vi "Cond Attr Get Clock.vi"(8 "error in (no error)":errorcluster, 11 "Cond Attr in":T2) -> (0 "error out":errorcluster, 2 "clock id":T1=enum."Monotonic", 3 "Cond Attr out":T2)   [LabVIEW 2016, in "Linux RT IPC.POSIX Threads.lvlib" / "Cond Attr.lvclass"]
doc: "Calls pthread_condattr_getclock() on the pthread cond attribute object encapsulated by Cond Attr.\n\nThis VI returns the current clock that the conditional variable is configured to use for timeout evaluation.\n\nRefer to online POSIX documentation for more information."
uses:
  Cond Attr.lvclass
  Controls/reference.ctl
  C:/Git/SourceTree/LinuxRT-IPC/Source/POSIX Threads/Classes/POSIX Thread Object/POSIX Thread Object.lvclass
  <vilib>/NI/NI Linux RT Utilities/Controls/Public/C Enums/clockid_t.ctl
  POSIX Thread Object/POSIX Thread Object.lvclass/POSIX Thread Object.ctl
  POSIX Thread Object/Private VIs/libpthread path.vi
  POSIX Thread Object/Private VIs/get pthread error.vi
  POSIX Thread Object/POSIX Thread Object.lvclass
  <vilib>/NI/NI Linux RT Utilities/Linux RT Utilities.lvlib
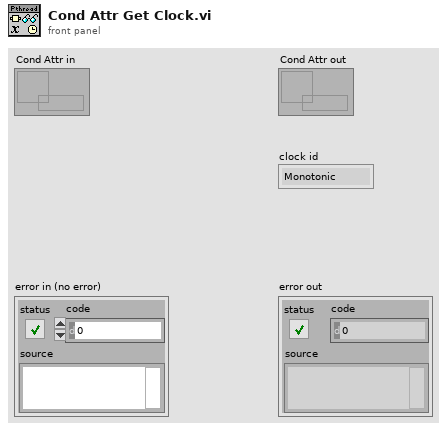
[diagram p1: front panel]
types:
  T1 = typedef "Linux RT Utilities.lvlib/clockid_t.ctl" = enum16{"Realtime", "Monotonic"}
  T2 = typedef "Linux RT IPC.POSIX Threads.lvlib/Cond Attr.lvclass/reference.ctl" = refnum<data-value>
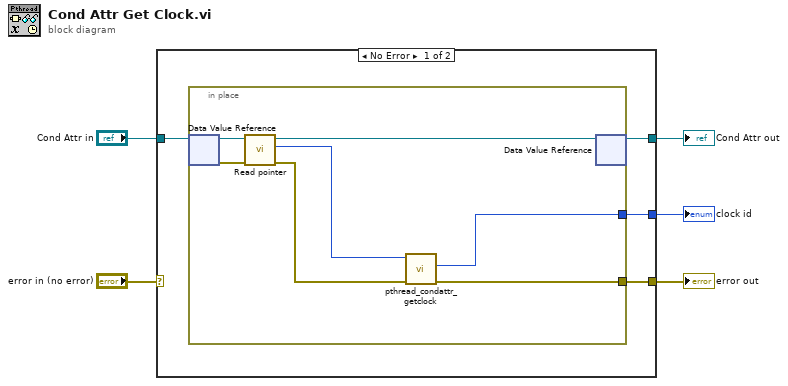
[diagram p0: block diagram]
diagram:
  n1 = case shown="No Error" "error in (no error)" {
    selector: "error in (no error)" -> [_ w18]
    tunnel: [w7 w18] -> w4
    tunnel: "Cond Attr in" -> [w9 w17]
    tunnel: [w8 w17] -> w2
    tunnel: [w6 _] -> w1
    frame No Error {
      n2 = in-place {
        in-place-border: [w12] -> w7
        in-place-border: [w10] -> w6
        n3 = in-place-dvr #1(w9) -> (w16:refnum<class "Cond Attr.lvclass">, w14:errorcluster)
        n4 = call "Read pointer.vi"("error in (no error)"=w14, "POSIX Thread Object in"=w16) -> ("error out"=w13:errorcluster, "pointer"=w11:u64, "POSIX Thread Object out"=w15:refnum<class "Cond Attr.lvclass">)  [unwired: 7 in]
        n5 = call "pthread_condattr_getclock.vi"("error in (no error)"=w13, "cond attr ptr in"=w11) -> ("error out"=w12:errorcluster, "clock id"=w10:T1)  [unwired: 7 in, 1 out]
        n6 = in-place-dvr #1(w15) -> (w8:T2)  [unwired: 1 out]
      }
    }
    frame Error {
    }
  }
  "Cond Attr out" <- w2
  "error out" <- w4
  "clock id" <- w1
